vi "AnalyzeGreyLevelOfDroplet.vi"(8 "error in (no error)":errorcluster, 10 "Bounding Box":cluster{"x":sgl, "y":sgl}[][](array[cluster]), 11 "Image In":T1(plugin-control)) -> (0 "error out":errorcluster, 2 "GreyLevelArray":dbl[](array[numeric]), 3 "Image Out":T1(plugin-control))   [LabVIEW 2013]
uses:
  <vilib>/Analysis/NI_AALBase.lvlib
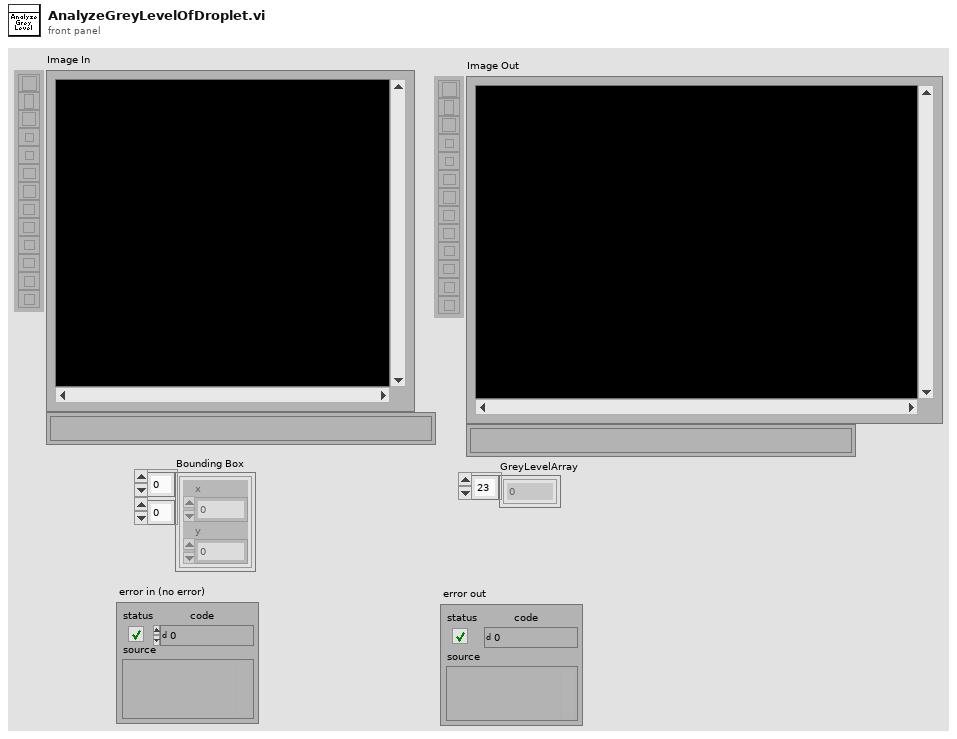
[diagram p1: front panel]
types:
  T1 = typedef "IMAQ Image.ctl" = refnum<image>
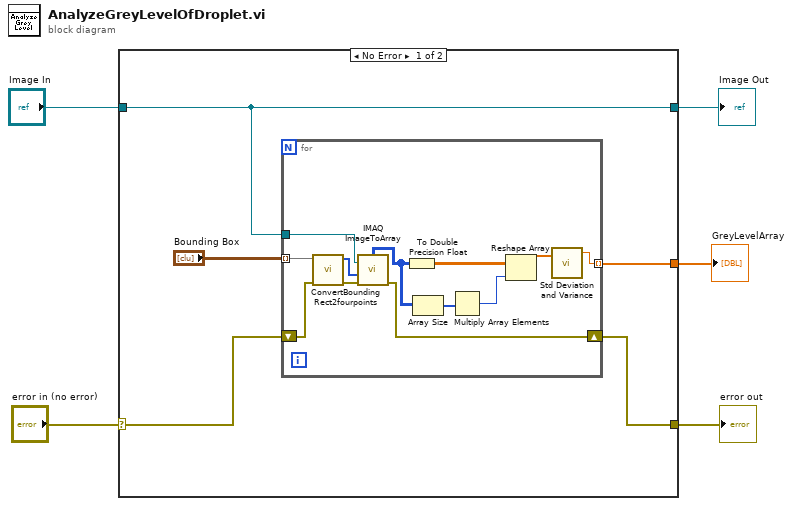
[diagram p0: block diagram]
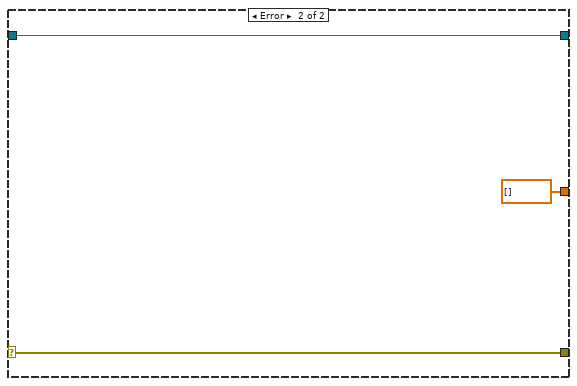
[diagram p2: hidden frame]
diagram:
  n1 = case shown="No Error" "error in (no error)" {
    selector: "error in (no error)" -> [w8 w25]
    tunnel: [w7 w25] -> w4
    tunnel: [w10 w24] -> w2
    tunnel: "Image In" -> [w10 w24]
    tunnel: [w6 dbl[] []] -> w1
    frame No Error {
      n2 = for {
        tunnel: w10 -> [w22]
        tunnel: "Bounding Box" -> [w20] mode=indexing
        shift-right: [w18] -> w7
        shift-left: w8 -> [w21]
        tunnel: [w11] -> w6 mode=indexing
        n3 = call "ConvertBoundingRect2fourpoints.vi"("Error In"=w21, "Bounding Box"=w20) -> ("Error Out"=w19:errorcluster, "Array"=w17:i32[])  [unwired: 8 in]
        n4 = call "IMAQ ImageToArray"("error in (no error)"=w19, "Optional Rectangle"=w17, "Image"=w22) -> ("error out"=w18:errorcluster, "Image Pixels (U8)"=w16:u8[][])  [unwired: 1 in, 3 out]
        n5 = To Double Precision Float(number=w16) -> (double precision float=w14:dbl[][])
        n6 = Array Size(array=w16) -> (size(s)=w15:i32[])
        n7 = Multiply Array Elements(1:w15) -> (0:w12:i32)
        n8 = Reshape Array(w14, w12) -> (w13:dbl[])
        n9 = call <vilib>:"Std Deviation and Variance.vi"("X"=w13) -> ("mean"=w11:dbl)  [unwired: 1 in, 2 out]
      }
    }
    frame Error {
    }
  }
  "error out" <- w4
  "Image Out" <- w2
  "GreyLevelArray" <- w1
